vi "JSONRPC Server.vi"(6 "LabVIEW Web Service":refnum<class "Web Service.lvclass">) -> ()   [LabVIEW 2015]
uses:
  <vilib>/wsapi/Web Service.lvclass
  Source/Classes/Request/Request.lvclass/Request.ctl
  Source/Classes/Request/Read method.vi
  Source/Classes/Request/Read params.vi
  Source/Classes/Server/Add Response (Result from Request).vi
  Source/Classes/Server/Add Response (Internal Error from Request).vi
  <vilib>/NI/JSON Support for LabVIEW/JSON Data Classes/JSON String/New JSON String.vi
  Source/Classes/Server/Add Response (Method Not Found from Request).vi
  Source/Classes/Server/Add Response (Server Error from Request).vi
  <vilib>/NI/JSON Support for LabVIEW/JSON Data Classes/JSON Datatype/JSON Null.lvclass
  Source/Classes/params/params.lvclass
  Source/Classes/Server/JSONRPC Server.lvclass
  Source/Classes/Request/Request.lvclass
  <vilib>/NI/JSON Support for LabVIEW/JSON Data Classes/JSON Helper/JSON Helper.lvclass
  <vilib>/NI/JSON Support for LabVIEW/JSON Data Classes/JSON String/JSON String.lvclass
panel:
  in  "error in (no error)":errorcluster
  out "error out":errorcluster
  # "Use the web service input terminal to call the VIs on the Service subpalette of the Web Services palette. Do not remove it from the connector pane unless you don't need access to the palette."
  # "Any additional terminals added to the connector pane of a startup VI will be ignored."
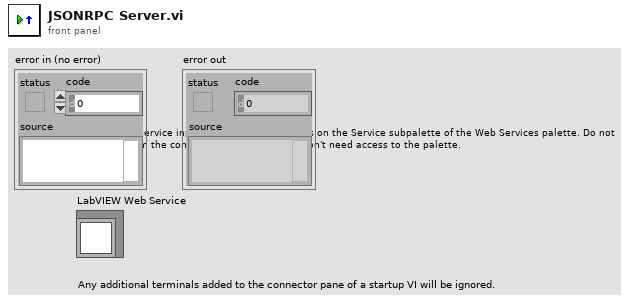
[diagram p1: front panel]
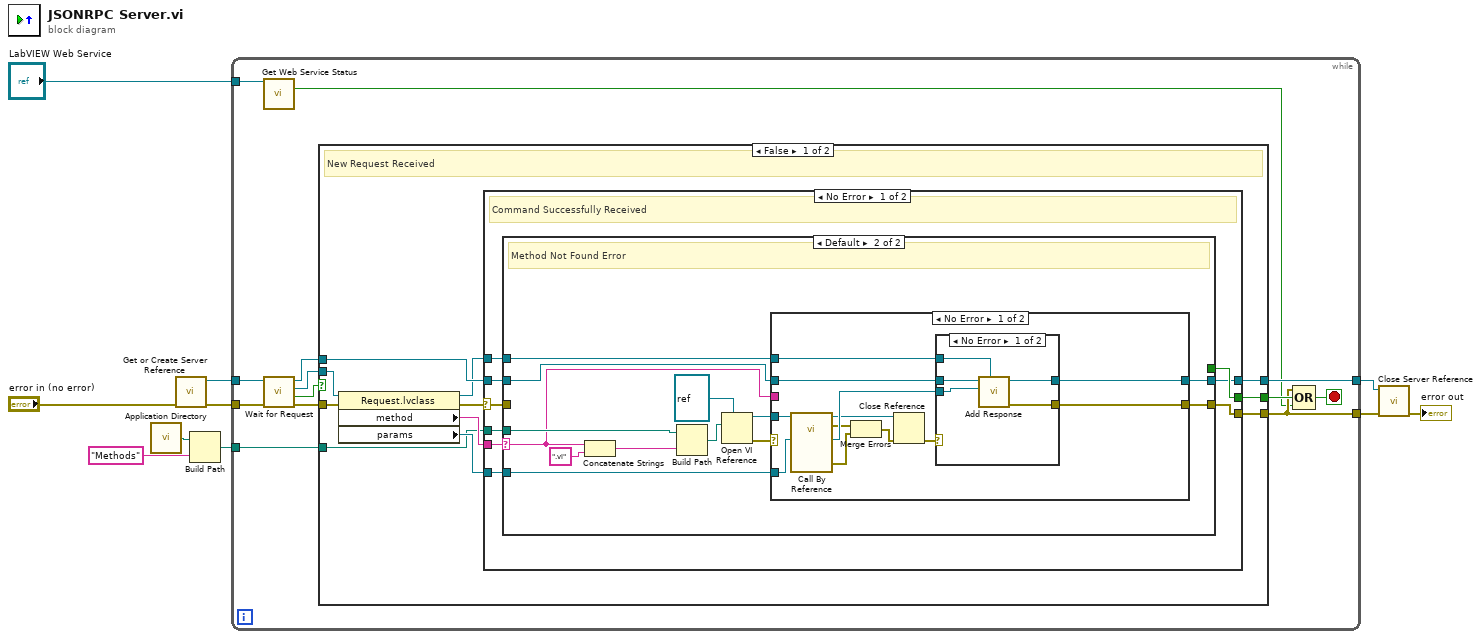
[diagram p0: block diagram]
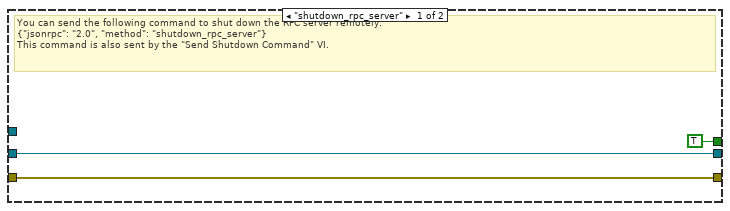
[diagram p2: hidden frame]
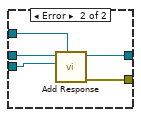
[diagram p3: hidden frame]
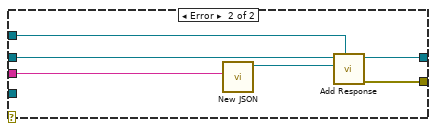
[diagram p4: hidden frame]
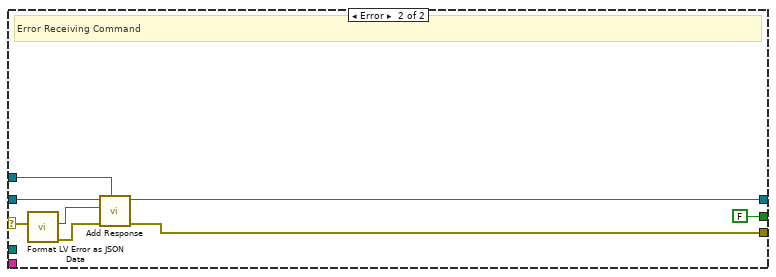
[diagram p5: hidden frame]
diagram:
  n1 = call <vilib>:"Application Directory.vi"() -> ("Application Directory"=w3:path)
  n2 = call "Get or Create Server Reference.vi"("error in (no error)"="error in (no error)") -> ("error out"=w9:errorcluster, "Server Out"=w10:refnum<class "JSONRPC Server.lvclass">)  [unwired: 9 in]
  n3 = Build Path(base path=w3, name or relative path="Methods") -> (appended path=w1:path)
  n4 = while {
    tunnel: w10 -> [w23]
    tunnel: w9 -> [w19]
    tunnel: [w15] -> w7
    tunnel: [w17] -> w8
    tunnel: "LabVIEW Web Service" -> [w13]
    tunnel: w1 -> [w11]
    stop <- w14 stop-if-true
    n5 = call <vilib>:"Get Web Service Status.vi"("LabVIEW Web Service"=w13) -> ("service stopping?"=w12:bool)  [unwired: 12 in, 2 out]
    n6 = call "Wait for Request.vi"("error in (no error)"=w19, "Server in"=w23) -> ("error out"=w18:errorcluster, "timed out?"=w20:bool, "Request"=w21:refnum<class "Request.lvclass">, "Server out"=w22:refnum<class "JSONRPC Server.lvclass">)  [unwired: 6 in]
    n7 = case shown="False" w20 {
      tunnel: w22 -> [w27 w96]
      tunnel: w21 -> [w34 _]
      tunnel: w18 -> [w31 w97]
      tunnel: [w29 w97] -> w15
      tunnel: [w28 _] -> w16
      tunnel: [w26 w96] -> w17
      tunnel: w11 -> [w24 _]
      frame False {
        # "New Request Received"
        n8 = property class="Request.lvclass"(reference=w34, error in=w31) -> (reference out=w25:refnum<class "Request.lvclass">, error out=w30:errorcluster, "method"=w33:string, "params"=w32:refnum<class "JSON Null.lvclass">)
        n9 = case shown="No Error" w30 {
          selector: w30 -> [w41 w89]
          tunnel: w33 -> [w43 _]
          tunnel: w32 -> [w42 _]
          tunnel: [w40 w92] -> w29
          tunnel: [w39 FALSE] -> w28
          tunnel: w27 -> [w38 w94]
          tunnel: [w37 w93] -> w26
          tunnel: w25 -> [w36 w95]
          tunnel: w24 -> [w35 _]
          frame No Error {
            # "Command Successfully Received"
            n10 = case shown="Default" w43 {
              selector: w43 -> [_ w49]
              tunnel: w42 -> [_ w53]
              tunnel: w41 -> [w45 _]
              tunnel: [w45 w57] -> w40
              tunnel: [TRUE _] -> w39
              tunnel: w38 -> [w44 w59]
              tunnel: [w44 w56] -> w37
              tunnel: w36 -> [_ w58]
              tunnel: w35 -> [_ w51]
              frame "shutdown_rpc_server" {
                # "You can send the following command to shut down the RPC server remotely:\n{\"jsonrpc\": \"2.0\", \"method\": \"shutdown_rpc_server\"}\nThis command is also sent by the \"Send Shutdown Command\" VI."
              }
              frame Default {
                # "Method Not Found Error"
                n11 = Concatenate Strings(w49, ".vi" ("string")) -> (w48:string)
                n12 = Build Path(base path=w51, name or relative path=w48) -> (appended path=w50:path)
                n13 = Open VI Reference(type specifier VI Refnum (for type only)=refnum<vi> refnum, vi path=w50) -> (vi reference=w54:refnum<vi>, error out=w52:errorcluster)  [unwired: 4 in]
                n14 = case shown="No Error" w52 {
                  tunnel: w59 -> [w71 w86]
                  tunnel: w58 -> [w70 w87]
                  tunnel: [w69 w84] -> w57
                  tunnel: [w68 w85] -> w56
                  tunnel: w54 -> [w67 _]
                  tunnel: w53 -> [w66 _]
                  tunnel: w49 -> [_ w83]
                  frame No Error {
                    n15 = call-by-ref "?"(reference=w67, "params"=w66) -> (reference out=w61:refnum<vi>, error out=w64:errorcluster, 0:"error out"=w63:errorcluster, "data"=w65:refnum<class "JSON Null.lvclass">)  [unwired: 10 in]
                    n16 = Merge Errors(w64, w63) -> (w62:errorcluster)
                    n17 = Close Reference(reference=w61, error in (no error)=w62) -> (error out=w60:errorcluster)
                    n18 = case shown="No Error" w60 {
                      tunnel: w71 -> [w76 w81]
                      tunnel: w70 -> [w75 w80]
                      tunnel: [w74 w79] -> w69
                      tunnel: [w73 w78] -> w68
                      tunnel: w65 -> [w72 w77]
                      frame No Error {
                        n19 = call-poly "Add Response.vi"("Request"=w75, "JSON in"=w72, "Server in"=w76) -> ("error out"=w74:errorcluster, "Server out"=w73:refnum<class "JSONRPC Server.lvclass">)  [unwired: 6 in, 1 out]
                      }
                      frame Error {
                        n20 = call-poly "Add Response.vi"("Request"=w80, "data"=w77, "Server in"=w81) -> ("error out"=w79:errorcluster, "Server out"=w78:refnum<class "JSONRPC Server.lvclass">)  [unwired: 6 in, 1 out]
                      }
                    }
                  }
                  frame Error {
                    n21 = call-poly <vilib>:"New JSON.vi"("value"=w83) -> ("JSON String out"=w82:refnum<class "JSON String.lvclass">)  [unwired: 9 in, 1 out]
                    n22 = call-poly "Add Response.vi"("Request"=w87, "data"=w82, "Server in"=w86) -> ("error out"=w84:errorcluster, "Server out"=w85:refnum<class "JSONRPC Server.lvclass">)  [unwired: 6 in, 1 out]
                  }
                }
              }
            }
          }
          frame Error {
            # "Error Receiving Command"
            n23 = call "Format LV Error as JSON Data.vi"("error in"=w89) -> ("error out"=w90:errorcluster, "Error Object Out"=w88:refnum<class "JSON Object.lvclass">)  [unwired: 9 in]
            n24 = call-poly "Add Response.vi"("Request"=w95, "error in (no error)"=w90, "data"=w88, "Server in"=w94) -> ("error out"=w92:errorcluster, "Server out"=w93:refnum<class "JSONRPC Server.lvclass">)  [unwired: 5 in, 1 out]
          }
        }
      }
      frame True {
        # "Timeout while waiting for new Requests"
      }
    }
    n25 = Compound Arithmetic op=OR(w15, w16, w12) -> (w14:bool)
  }
  n26 = call-dynamic "Close Server Reference.vi"("error in (no error)"=w7, "Server in"=w8) -> ("error out"=→"error out":errorcluster)  [unwired: 9 in]
